vi "v1.vi"   [LabVIEW 2023]
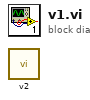
[diagram p0: block diagram]
diagram:
  n1 = call "v2.vi"() -> ()  [unwired: 12 in]
